vi "Drop Protobuf To Field Converter SubVI.vi"(8 "error in (no error)":errorcluster, 10 "Owner VI in":refnum<vi>, 11 "Library":refnum<vi>) -> (0 "error out":errorcluster, 1 "SubVI out":refnum<vi>, 2 "Owner VI out":refnum<vi>, 3 "Library out":refnum<vi>)   [LabVIEW 2019, in "gRPC Template Creation Utility.lvlib"]
uses:
  gRPC Template Creation Utility.lvlib
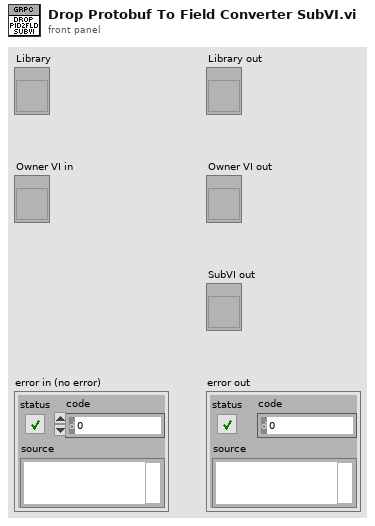
[diagram p1: front panel]
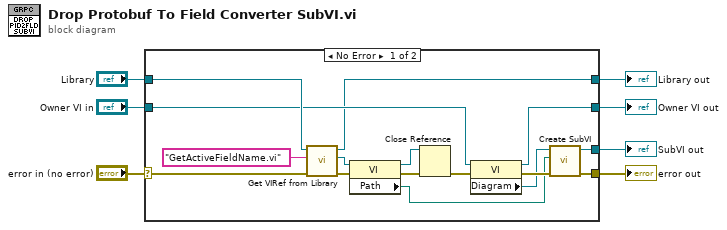
[diagram p0: block diagram]
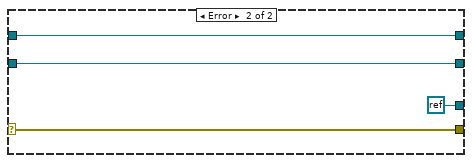
[diagram p2: hidden frame]
diagram:
  n1 = case shown="No Error" "error in (no error)" {
    selector: "error in (no error)" -> [w13 w27]
    tunnel: [w23 refnum<k0> refnum] -> w7
    tunnel: [w22 w27] -> w6
    tunnel: "Library" -> [w17 w26]
    tunnel: "Owner VI in" -> [w15 w24]
    tunnel: [w14 w24] -> w3
    tunnel: [w12 w26] -> w1
    frame No Error {
      n2 = call "Get VIRef from Library.vi"("error in (no error)"=w13, "item name"="GetActiveFieldName.vi" ("format string"), "library in"=w17) -> ("error out"=w19:errorcluster, "vi"=w18:refnum<vi>, "library out"=w12:refnum<vi>)  [unwired: 5 in, 1 out]
      n3 = property class="VI"(reference=w18, error in=w19) -> (reference out=w9:refnum<vi>, error out=w10:errorcluster, "Path"=w20:path)
      n4 = Close Reference(reference=w9, error in (no error)=w10) -> (error out=w8:errorcluster)
      n5 = property class="VI"(reference=w15, error in=w8) -> (reference out=w14:refnum<vi>, error out=w21:errorcluster, "Diagram"=w16:refnum<vi>)
      n6 = call "Create SubVI.vi"("error in (no error)"=w21, "Path"=w20, "Diagram in"=w16) -> ("error out"=w22:errorcluster, "subVI refnum"=w23:refnum<vi>)  [unwired: 7 in]
    }
    frame Error {
    }
  }
  "SubVI out" <- w7
  "error out" <- w6
  "Library out" <- w1
  "Owner VI out" <- w3
